vi "VI Server_Close VI Controls RefsWithoutError.vi"(8 "error in (no error)":errorcluster, 11 "VI Server Cluster":T1) -> (0 "error out":errorcluster)   [LabVIEW 2020, in "VI Server Toolkit LV2013.lvlib"]
doc: "Closes controls/indicators and VI references.\nTypically used at a calling VI exit.\n\n<B>NOTE</B>:\nErrors generated while closing references are discarded."
uses:
  VI Server Toolkit LV2013.lvlib
  VI Server_TypeDefs/VI Server_RefsCluster.ctl
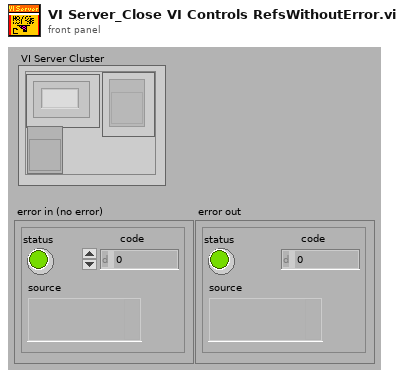
[diagram p1: front panel]
types:
  T1 = typedef "VI Server_RefsCluster.ctl" = cluster{"Labels":string[], "Refs":refnum<vi>[], "VI Ref":refnum<vi>}
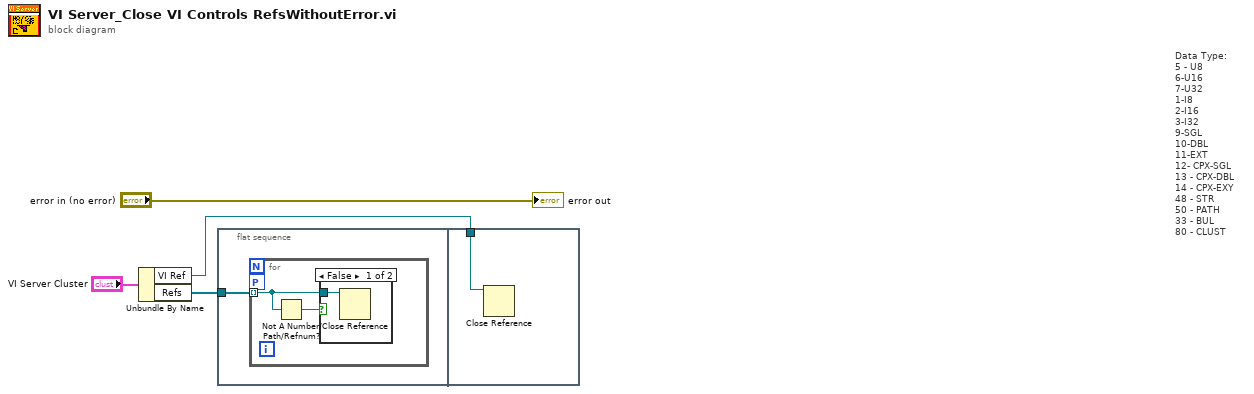
[diagram p0: block diagram]
diagram:
  # "Data Type:\n5 - U8\n6-U16\n7-U32\n1-I8\n2-I16\n3-I32\n9-SGL\n10-DBL\n11-EXT\n12- CPX-SGL\n13 - CPX-DBL\n14 - CPX-EXY\n48 - STR\n50 - PATH\n33 - BUL\n80 - CLUST"
  n1 = Unbundle By Name("VI Server Cluster") -> ("VI Ref"=w1:refnum<vi>, "Refs"=w3:refnum<vi>[])
  n2 = flat-sequence {
    tunnel: w3 -> [w5]
    tunnel: w1 -> [w9]
    frame #0 {
      n3 = for {
        tunnel: w5 -> [w6] mode=indexing
        workers-P: _ -> [_]
        n4 = Not A Number/Path/Refnum?(number/path/refnum=w6) -> (NaN/Path/Refnum?=w7:bool)
        n5 = case shown="False" w7 {
          tunnel: w6 -> [w8 _]
          frame False {
            n6 = Close Reference(reference=w8) -> ()  [unwired: 1 in, 1 out]
          }
          frame True {
          }
        }
      }
    }
    frame #1 {
      n7 = Close Reference(reference=w9) -> ()  [unwired: 1 in, 1 out]
    }
  }
  "error out" <- "error in (no error)"
